vi "Path.vi"(11 "WebSocket Client in":refnum<class "WebSocket Client.lvclass">) -> (2 "Path":string, 3 "WebSocket Client out":refnum<class "WebSocket Client.lvclass">)   [LabVIEW 2020, in "HTTP Server.lvlib" / "WebSocket Client.lvclass"]
uses:
  WebSocket Client.lvclass
  WebSocket Client.lvclass/WebSocket Client.ctl
  lv-http-util/HTTP Utils/Request/Request.lvclass
  lv-uri/URI/URI/URI.lvclass
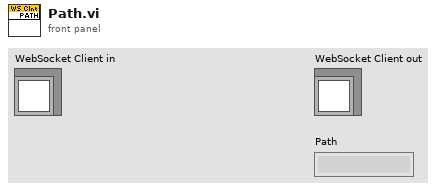
[diagram p1: front panel]
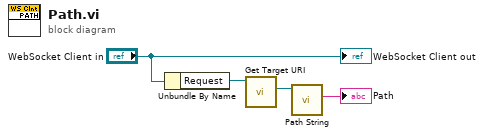
[diagram p0: block diagram]
diagram:
  n1 = Unbundle By Name("WebSocket Client in") -> ("Request"=w3:refnum<class "Request.lvclass">)
  n2 = call "Get Target URI.vi"("Request in"=w3) -> ("Target URI"=w2:refnum<class "URI.lvclass">)  [unwired: 8 in, 2 out]
  n3 = call "Path String.vi"("URI in"=w2) -> ("Path String"=→"Path":string)  [unwired: 9 in, 1 out]
  "WebSocket Client out" <- "WebSocket Client in"
